vi "stateSwitch.vi"(8 "disable":bool, 11 "enable":bool) -> (3 "state":bool)   [LabVIEW 2016]
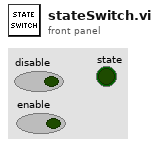
[diagram p1: front panel]
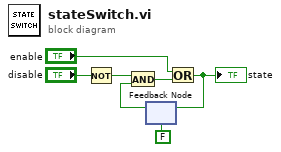
[diagram p0: block diagram]
diagram:
  n1 = Not(x="disable") -> (.not. x?=w3:bool)
  n2 = feedback #1(FALSE) -> (w4:bool)
  n3 = And(x=w3, y=w4) -> (x .and. y?=w6:bool)
  n4 = Or(x="enable", y=w6) -> (x .or. y?=w5:bool)
  "state" <- w5
  n5 = feedback-in #1(w5) -> ()
